vi "Search_Element.vi"(0 "Queue in":refnum<queue>, 1 "String":string, 2 "error in (no error)":errorcluster) -> (3 "cluster":cluster{"Test Name":string, "File Path":path}, 4 "Numeric":i32, 5 "Boolean":bool, 6 "error out":errorcluster)   [LabVIEW 2018]
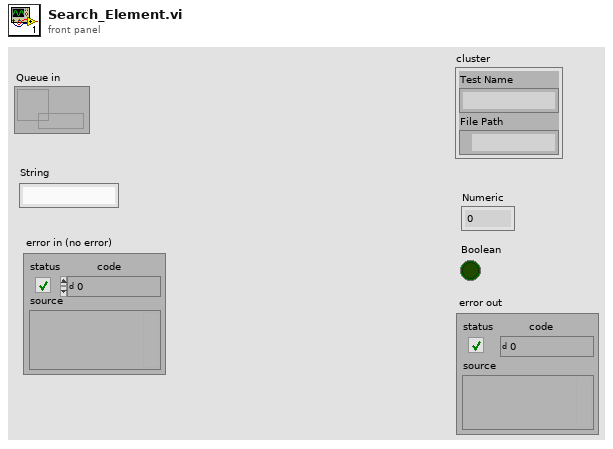
[diagram p1: front panel]
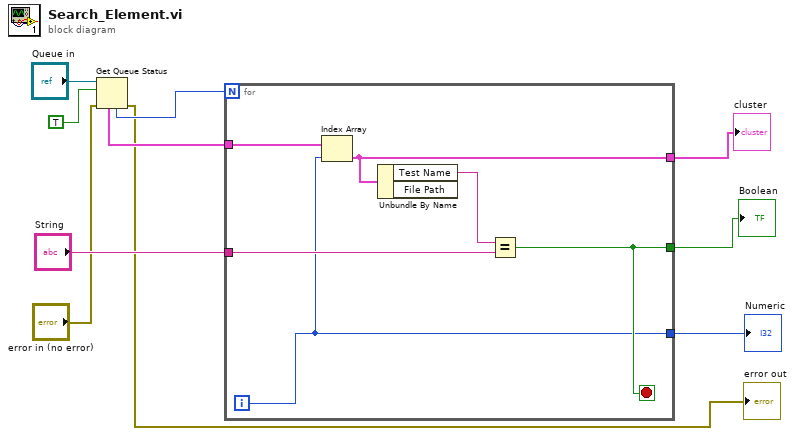
[diagram p0: block diagram]
diagram:
  n1 = Get Queue Status(queue="Queue in", return elements? (F)=TRUE, error in (no error)="error in (no error)") -> (error out=→"error out":errorcluster, # elements in queue=w8:i32, elements=w7:cluster{"Test Name":string, "File Path":path}[])  [unwired: 5 out]
  n2 = for {
    N: w8 -> [_]
    tunnel: w7 -> [w16]
    tunnel: "String" -> [w15]
    tunnel: [w13] -> w5
    tunnel: [w12] -> w4
    tunnel: [w11] -> w1
    i -> [w12]
    stop <- w13 stop-if-true
    n3 = Index Array(array=w16, index=w12) -> (element=w11:cluster{"Test Name":string, "File Path":path})
    n4 = Unbundle By Name(w11) -> ("Test Name"=w14:string)  [unwired: 1 out]
    n5 = Equal?(x=w14, y=w15) -> (x = y?=w13:bool)
  }
  "Boolean" <- w5
  "Numeric" <- w4
  "cluster" <- w1
